vi "Ticks to Rotations (Steer).vi"(11 "Steer Angles (ticks)":T1) -> (3 "Steer Angles (rotations)":T1)   [LabVIEW 2020]
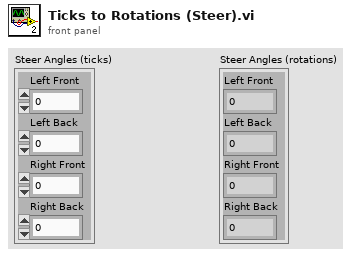
[diagram p1: front panel]
types:
  T1 = cluster{"Left Front":dbl, "Left Back":dbl, "Right Front":dbl, "Right Back":dbl}
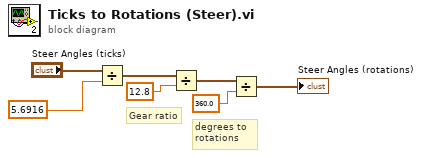
[diagram p0: block diagram]
diagram:
  # "degrees to rotations"
  # "Gear ratio"
  n1 = Divide(x="Steer Angles (ticks)", y=5.6916 ("Scale Factor")) -> (x/y=w7:T1)
  n2 = Divide(x=w7, y=12.8) -> (x/y=w3:T1)
  n3 = Divide(x=w3, y=360.0) -> (x/y=→"Steer Angles (rotations)":T1)
